vi "Write to ThingSpeak.vi"(1 "error in":errorcluster, 2 "Temp Value":dbl, 3 "Field":i32, 4 "API Key":string) -> (0 "error out":errorcluster)   [LabVIEW 2022 SP3]
uses:
  <vilib>/httpClient/LabVIEWHTTPClient.lvlib
panel:
  out "URL":string
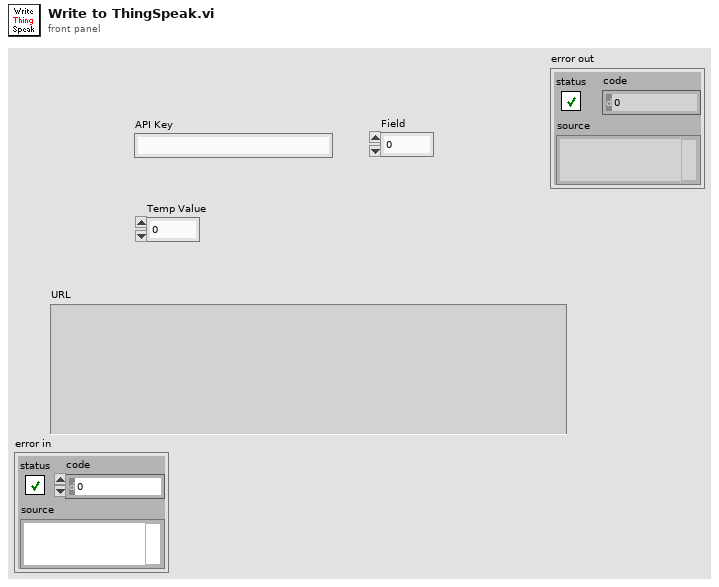
[diagram p1: front panel]
types:
  T1 = typedef "LabVIEWHTTPClient.lvlib/ClientHandle.ctl" = refnum<k1>
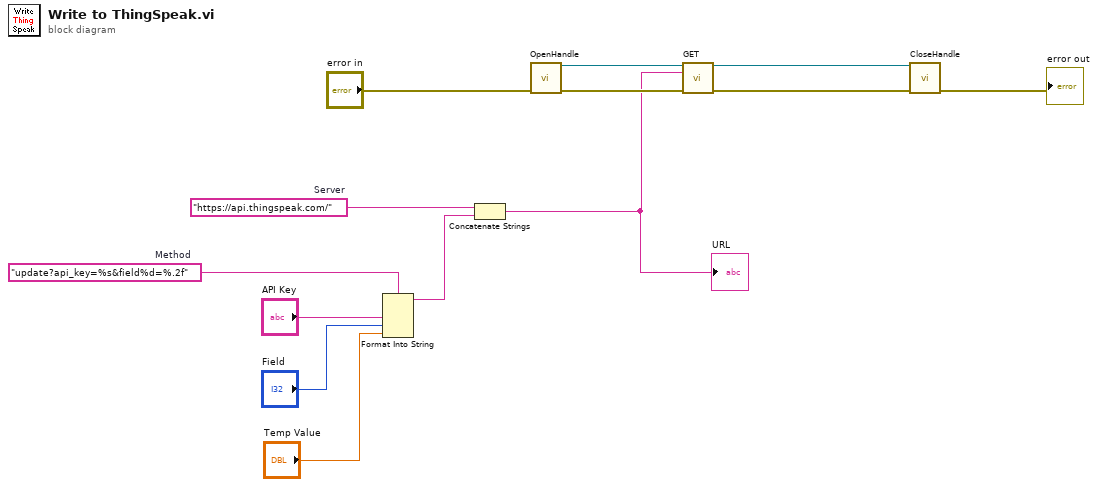
[diagram p0: block diagram]
diagram:
  w8 = "update?api_key=%s&field%d=%.2f"  # Method
  w9 = "https://api.thingspeak.com/"  # Server
  n1 = Format Into String(format string=w8, "API Key", "Field", "Temp Value") -> (resulting string=w4:string)  [unwired: 2 in, 1 out]
  n2 = Concatenate Strings "Concatenate Strings"(w9, w4) -> (w3:string)
  "URL" <- w3
  n3 = call <vilib>:"OpenHandle.vi"("error in (no error)"="error in") -> ("client handle out"=w13:T1, "error out"=w12:errorcluster)  [unwired: 13 in]
  n4 = call <vilib>:"GET.vi"("client handle"=w13, "url"=w3, "error in (no error)"=w12) -> ("client handle out"=w10:T1, "error out"=w11:errorcluster)  [unwired: 9 in, 2 out]
  n5 = call <vilib>:"CloseHandle.vi"("client handle"=w10, "error in (no error)"=w11) -> ("error out"=→"error out":errorcluster)  [unwired: 13 in]
